vi "CC Script Parse.vi"(8 "error in (no error)":errorcluster, 11 "Script text":string="DefineObject \"Test\" Type=Standard,PositionType=RA-DEC,RA=14:25:33.123,DEC=090:15:22.110,muRA=0.000000,muDEC=0.000000,Epoch=0.000000,xi=1.000000,eta=2.000000,dRA=3.000000,dDEC=4.000000\nDefineExposure \"Standard\" Number=1,ReadoutGroups=1,ReadoutsperGroup=2,TimeBetweenGroups=10.000000,TimeBetweenReadouts=10.000000\nDefineDithering Random \"\" Count=1,Radius=1FocusMoveAbsolute Motor=1,Position=23452\nFocusMoveRelative Motor=1,Distance=23452\nAcquireImage Object=\"Test\",Exposure=\"Standard\",Dithering=\"Random\"\nFocusSetHome Motor=1\nFocusMoveRelative Motor=1,Distance=23452\nFocusMoveRelative Motor=1,Distance=23452\nTelescopeFocusHome\nTelescopeFocusMove Position=-0.123\n") -> (0 "error out":errorcluster, 1 "Syntax Errors":string, 2 "Script Ok?":bool, 3 "Script steps":T1[](array[typedef]))   [LabVIEW 2021]
uses:
  typedefs/CC Script Step.ctl
  typedefs/CC enum Script Action.ctl
  <vilib>/regexp/Match Regular Expression.xnode
panel:
  out "Errors":errorcluster[](array[cluster])
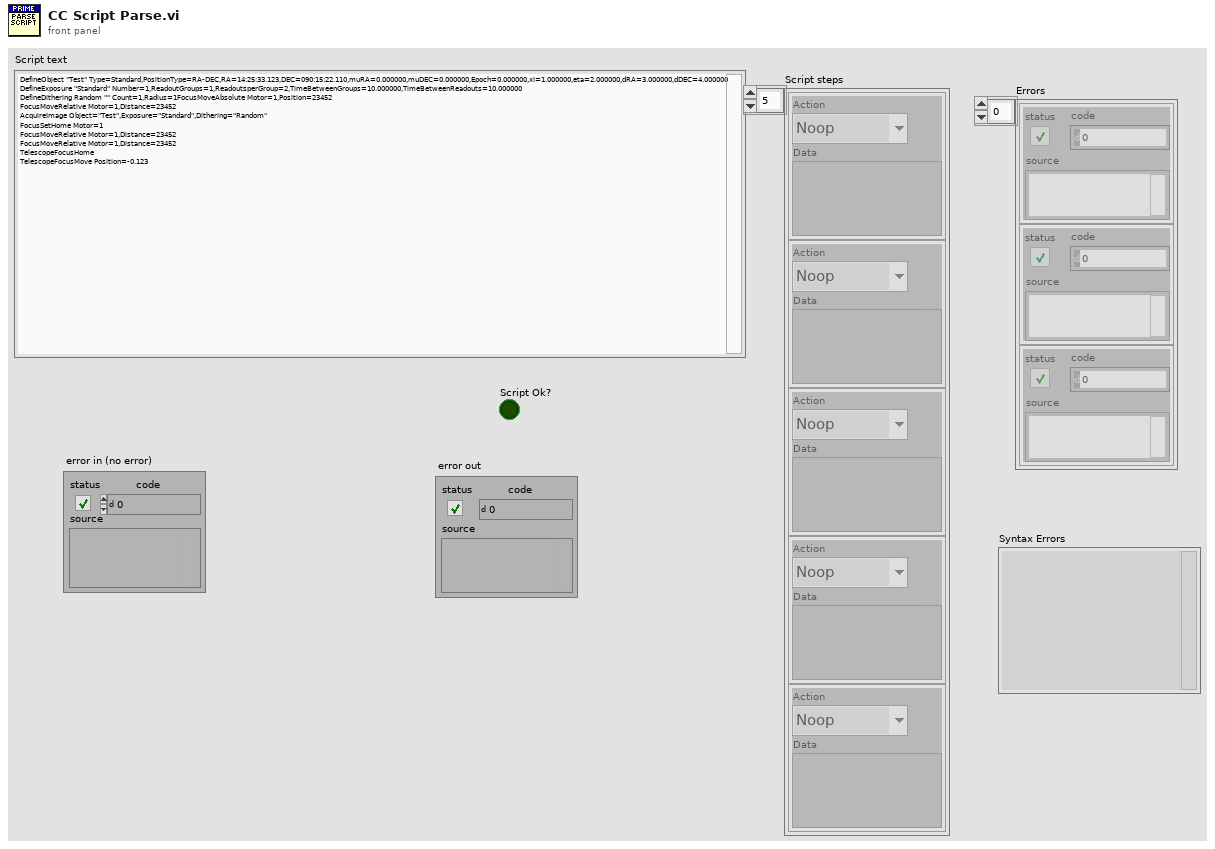
[diagram p1: front panel]
types:
  T1 = typedef "CC Script Step.ctl" = cluster{"Action":T2, "Data":variant}
  T2 = typedef "CC enum Script Action.ctl" = enum16{"Noop", "Define Object", "Define Exposure", "Define Dithering", "Acquire Images", "Set Filter Wheel", "Telescope Home", "Telescope Move", "Telescope RA DEC", "Focus Move Relative", "Focus Move Absolute", "Focus Set Home", "Macro", "Pause", "Ask User", "Define Random Dither"}
  T3 = typedef "CC cluster Object.ctl" = cluster{"Object":cluster{"Name":string}, "Sidereal Rate":T4, "RA and DEC":T5, "muRA muDEC Epoch":T6, "Offsets":T7}
  T4 = typedef "CC cluster sidereal rate.ctl" = cluster{"dRA":dbl, "dDEC":dbl}
  T5 = typedef "CC cluster RA and DEC.ctl" = cluster{"RA":dbl, "DEC":dbl}
  T6 = typedef "cc cluster muRA muDEC.ctl" = cluster{"muRA":dbl, "muDEC":dbl, "Epoch":dbl}
  T7 = typedef "CC cluster Telescope Offsets.ctl" = cluster{"RA":dbl, "DEC":dbl, "ROT":dbl}
  T8 = typedef "CC cluster Exposure.ctl" = cluster{"Mode":T9, "Integration Time":dbl, "Name":string, "Images":i32}
  T9 = typedef "Detector enum Detector Integration Mode.ctl" = enum16{"SSR", "CDS", "MEAN", "MEDIAN", "MODE", "MIIN", "MAX"}
  T10 = typedef "CC Dithering.ctl" = cluster{"Name":string, "Dithering Offsets":T11}
  T11 = typedef "CC cluster Offset Dithering.ctl" = cluster{"Offsets":T12[]}
  T12 = typedef "CC Dithering Offsets.ctl" = cluster{"DEC":dbl, "RA":dbl}
  T13 = typedef "CC cluster Random Dithering.ctl" = cluster{"Count":i32, "Radius":dbl, "Name":string}
  T14 = typedef "CC cluster Acquire Parameters.ctl" = cluster{"Object":string, "Exposure":string, "Dithering":string}
  T15 = typedef "CC cluster Filter Wheel Parameters.ctl" = cluster{"Wheel":i32, "Filter":i32}
  T16 = typedef "Focus cluster MoveFocus Command Parameters.ctl" = cluster{"Motor":i32, "Position":i32}
  T17 = typedef "CC cluster Pause Parameters.ctl" = cluster{"Time (s)":dbl}
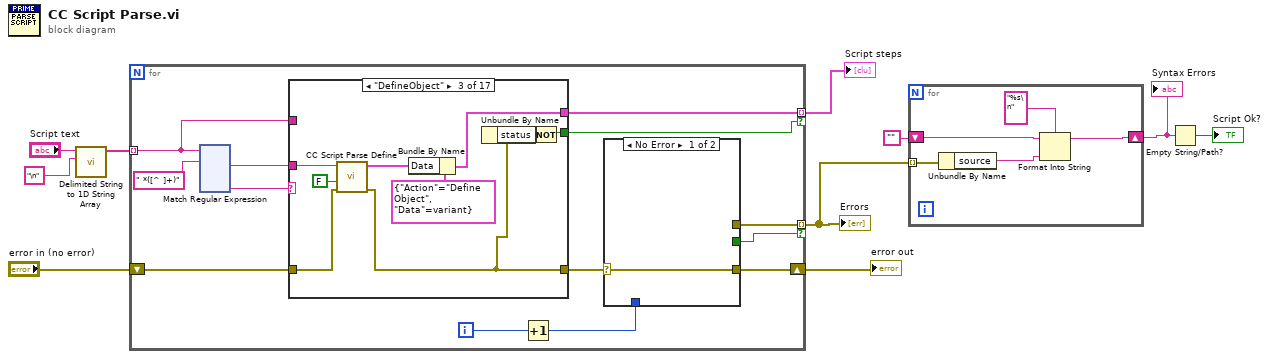
[diagram p0: block diagram]
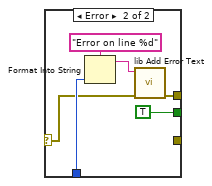
[diagram p2: hidden frame]
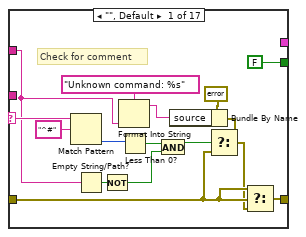
[diagram p3: hidden frame]
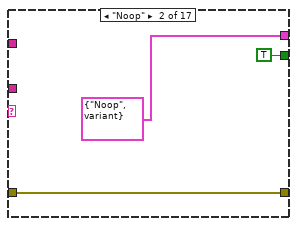
[diagram p4: hidden frame]
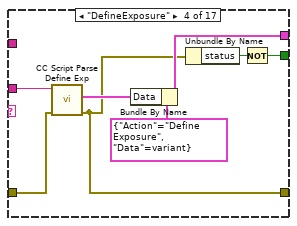
[diagram p5: hidden frame]
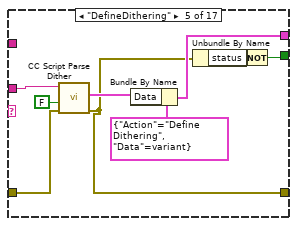
[diagram p6: hidden frame]
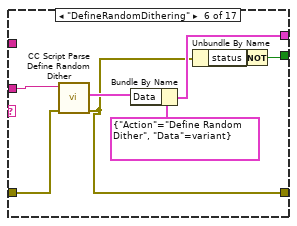
[diagram p7: hidden frame]
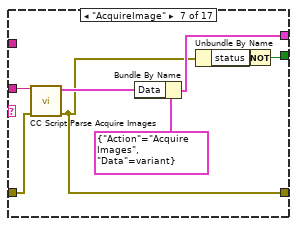
[diagram p8: hidden frame]
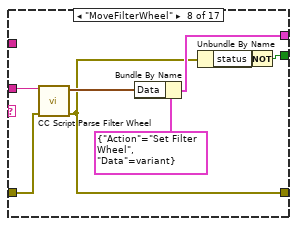
[diagram p9: hidden frame]
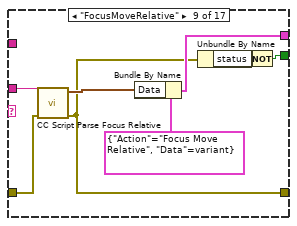
[diagram p10: hidden frame]
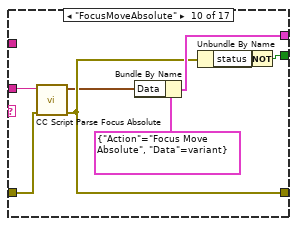
[diagram p11: hidden frame]
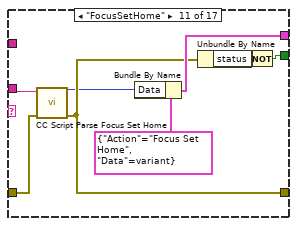
[diagram p12: hidden frame]
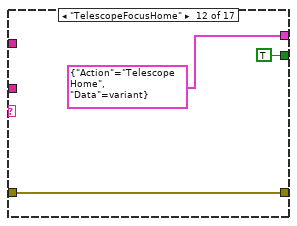
[diagram p13: hidden frame]
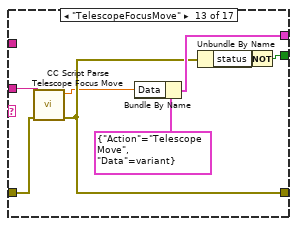
[diagram p14: hidden frame]
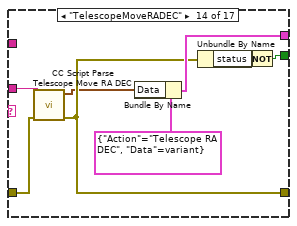
[diagram p15: hidden frame]
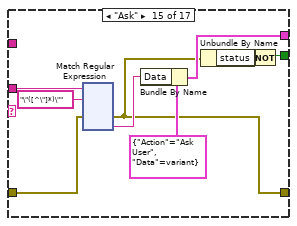
[diagram p16: hidden frame]
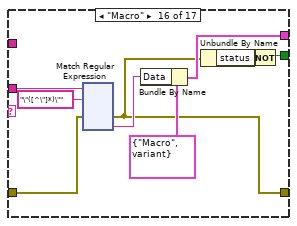
[diagram p17: hidden frame]
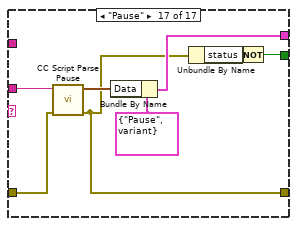
[diagram p18: hidden frame]
diagram:
  n1 = call <vilib>:"Delimited String to 1D String Array.vi"("delimiter"="\n", "delimited string"="Script text") -> ("string array"=w9:string[])  [unwired: 9 in]
  n2 = for {
    tunnel: w9 -> [w15] mode=indexing
    shift-right: [w19] -> w6
    shift-left: "error in (no error)" -> [w21]
    tunnel: [w17] -> w4 mode=indexing if=w13
    tunnel: [w14] -> w5 mode=indexing if=w12
    i -> [w18]
    n3 = xnode "Match Regular Expression"("input string"=w15, "regular expression"=" *([^ ]+)") -> ("after match"=w22:string, "submatch 1"=w11:string)  [unwired: 4 in, 4 out]
    n4 = case shown="\"DefineObject\"" w11 {
      selector: w11 -> [w36 _ _ _ _ _ _ _ _ _ _ _ _ _ _ _ _]
      tunnel: w22 -> [_ _ w58 w65 w71 w79 w90 w98 w103 w108 w119 _ w130 w138 w151 w279 w405]
      tunnel: [_ T1 {"Action"=enum."Noop", "Data"=variant} ("Cluster") w53 w62 w74 w82 w87 w95 w106 w114 w122 T1 {"Action"=enum."Telescope Home", "Data"=variant} ("Cluster") w133 w141 w146 w274 w402] -> w14
      tunnel: w21 -> [w39 w49 w56 w63 w70 w78 w88 w96 w102 w111 w118 w124 w129 w137 w147 w275 w403]
      tunnel: [w37 w49 w52 w60 w68 w76 w85 w93 w100 w110 w117 w124 w128 w136 w144 w272 w400] -> w20
      tunnel: w15 -> [w34 _ _ _ _ _ _ _ _ _ _ _ _ _ _ _ _]
      tunnel: [FALSE TRUE w50 w59 w72 w80 w84 w92 w104 w112 w120 TRUE w131 w139 w143 w271 w399] -> w12
      frame "", Default {
        # "Check for comment"
        n5 = Match Pattern(string=w36, regular expression="^#") -> (offset past match=w42:i32)  [unwired: 1 in, 3 out]
        n6 = Empty String/Path?(string/path=w34) -> (empty?=w32:bool)
        n7 = Not(x=w32) -> (.not. x?=w31:bool)
        n8 = Format Into String(format string="Unknown command: %s", w34) -> (resulting string=w43:string)  [unwired: 2 in, 1 out]
        n9 = Less Than 0?(x=w42) -> (x < 0?=w40:bool)
        n10 = And(x=w40, y=w31) -> (x .and. y?=w33:bool)
        n11 = Bundle By Name(cluster=errorcluster {"status"=TRUE, "code"=5000, "source"=""} ("error out"), "source"=w43) -> (w41:errorcluster)
        n12 = Select(t=w41, s=w33, f=w39) -> (s? t:f=w38:errorcluster)
        n13 = Select(t=w39, s=w39, f=w38) -> (s? t:f=w37:errorcluster)
      }
      frame "Noop" {
      }
      frame "DefineObject" {
        n14 = call "CC Script Parse Define.vi"("error in (no error)"=w56, "To String?"=FALSE, "DefineObject Parameters"=w58) -> ("error out"=w52:errorcluster, "Object out"=w54:T3)  [unwired: 5 in, 2 out]
        n15 = Bundle By Name(cluster=T1 {"Action"=enum."Define Object", "Data"=variant} ("Cluster"), "Data"=w54) -> (w53:T1)
        n16 = Unbundle By Name(w52) -> ("status"=w51:bool)
        n17 = Not(x=w51) -> (.not. x?=w50:bool)
      }
      frame "DefineExposure" {
        n18 = call "CC Script Parse Define Exp.vi"("error in (no error)"=w63, "DefineExp Parameters"=w65) -> ("error out"=w60:errorcluster, "Exposure"=w64:T8)  [unwired: 6 in, 2 out]
        n19 = Bundle By Name(cluster=T1 {"Action"=enum."Define Exposure", "Data"=variant} ("Cluster"), "Data"=w64) -> (w62:T1)
        n20 = Unbundle By Name(w60) -> ("status"=w61:bool)
        n21 = Not(x=w61) -> (.not. x?=w59:bool)
      }
      frame "DefineDithering" {
        n22 = call "CC Script Parse Dither.vi"("error in (no error)"=w70, "To String?"=FALSE, "Dither Parameters"=w71) -> ("error out"=w68:errorcluster, "Dithering out"=w69:T10)  [unwired: 6 in, 1 out]
        n23 = Bundle By Name(cluster=T1 {"Action"=enum."Define Dithering", "Data"=variant} ("Cluster"), "Data"=w69) -> (w74:T1)
        n24 = Unbundle By Name(w68) -> ("status"=w73:bool)
        n25 = Not(x=w73) -> (.not. x?=w72:bool)
      }
      frame "DefineRandomDithering" {
        n26 = call "CC Script Parse Define Random Dither.vi"("error in (no error)"=w78, "Dither Parameters"=w79) -> ("error out"=w76:errorcluster, "Random Dither out"=w77:T13)  [unwired: 7 in, 1 out]
        n27 = Bundle By Name(cluster=T1 {"Action"=enum."Define Random Dither", "Data"=variant} ("Cluster"), "Data"=w77) -> (w82:T1)
        n28 = Unbundle By Name(w76) -> ("status"=w81:bool)
        n29 = Not(x=w81) -> (.not. x?=w80:bool)
      }
      frame "AcquireImage" {
        n30 = call "CC Script Parse Acquire Images.vi"("error in (no error)"=w88, "DefineObject Parameters"=w90) -> ("error out"=w85:errorcluster, "Acquire Parameters"=w89:T14)  [unwired: 7 in, 1 out]
        n31 = Bundle By Name(cluster=T1 {"Action"=enum."Acquire Images", "Data"=variant} ("Cluster"), "Data"=w89) -> (w87:T1)
        n32 = Unbundle By Name(w85) -> ("status"=w86:bool)
        n33 = Not(x=w86) -> (.not. x?=w84:bool)
      }
      frame "MoveFilterWheel" {
        n34 = call "CC Script Parse Filter Wheel.vi"("error in (no error)"=w96, "DefineObject Parameters"=w98) -> ("error out"=w93:errorcluster, "Filter Wheel Parameters"=w97:T15)  [unwired: 7 in, 1 out]
        n35 = Bundle By Name(cluster=T1 {"Action"=enum."Set Filter Wheel", "Data"=variant} ("Cluster"), "Data"=w97) -> (w95:T1)
        n36 = Unbundle By Name(w93) -> ("status"=w94:bool)
        n37 = Not(x=w94) -> (.not. x?=w92:bool)
      }
      frame "FocusMoveRelative" {
        n38 = call "CC Script Parse Focus Relative.vi"("error in (no error)"=w102, "DefineObject Parameters"=w103) -> ("error out"=w100:errorcluster, "Filter Wheel parameters in"=w101:T16)  [unwired: 7 in, 1 out]
        n39 = Bundle By Name(cluster=T1 {"Action"=enum."Focus Move Relative", "Data"=variant} ("Cluster"), "Data"=w101) -> (w106:T1)
        n40 = Unbundle By Name(w100) -> ("status"=w105:bool)
        n41 = Not(x=w105) -> (.not. x?=w104:bool)
      }
      frame "FocusMoveAbsolute" {
        n42 = call "CC Script Parse Focus Absolute.vi"("error in (no error)"=w111, "FocusMoveAbsolute Parameters"=w108) -> ("error out"=w110:errorcluster, "Filter Wheel parameters in"=w109:T16)  [unwired: 7 in, 1 out]
        n43 = Bundle By Name(cluster=T1 {"Action"=enum."Focus Move Absolute", "Data"=variant} ("Cluster"), "Data"=w109) -> (w114:T1)
        n44 = Unbundle By Name(w110) -> ("status"=w113:bool)
        n45 = Not(x=w113) -> (.not. x?=w112:bool)
      }
      frame "FocusSetHome" {
        n46 = call "CC Script Parse Focus Set Home.vi"("error in (no error)"=w118, "DefineObject Parameters"=w119) -> ("error out"=w117:errorcluster, "Set Home Parm"=w116:i32)  [unwired: 7 in, 1 out]
        n47 = Bundle By Name(cluster=T1 {"Action"=enum."Focus Set Home", "Data"=variant} ("Cluster"), "Data"=w116) -> (w122:T1)
        n48 = Unbundle By Name(w117) -> ("status"=w121:bool)
        n49 = Not(x=w121) -> (.not. x?=w120:bool)
      }
      frame "TelescopeFocusHome" {
      }
      frame "TelescopeFocusMove" {
        n50 = call "CC Script Parse Telescope Focus Move.vi"("error in (no error)"=w129, "Telescope Move Parameters"=w130) -> ("error out"=w128:errorcluster, "Telescope Move Pos"=w127:dbl)  [unwired: 7 in, 1 out]
        n51 = Bundle By Name(cluster=T1 {"Action"=enum."Telescope Move", "Data"=variant} ("Cluster"), "Data"=w127) -> (w133:T1)
        n52 = Unbundle By Name(w128) -> ("status"=w132:bool)
        n53 = Not(x=w132) -> (.not. x?=w131:bool)
      }
      frame "TelescopeMoveRADEC" {
        n54 = call "CC Script Parse Telescope Move RA DEC.vi"("error in (no error)"=w137, "Telescope Move Parameters"=w138) -> ("error out"=w136:errorcluster, "RA and DEC"=w135:T5)  [unwired: 7 in, 1 out]
        n55 = Bundle By Name(cluster=T1 {"Action"=enum."Telescope RA DEC", "Data"=variant} ("Cluster"), "Data"=w135) -> (w141:T1)
        n56 = Unbundle By Name(w136) -> ("status"=w140:bool)
        n57 = Not(x=w140) -> (.not. x?=w139:bool)
      }
      frame "Ask" {
        n58 = xnode "Match Regular Expression"("input string"=w151, "regular expression"="\"([^\"]*)\"", "error in"=w147) -> ("error out"=w144:errorcluster, "submatch 1"=w148:string)  [unwired: 3 in, 4 out]
        n59 = Bundle By Name(cluster=T1 {"Action"=enum."Ask User", "Data"=variant} ("Cluster"), "Data"=w148) -> (w146:T1)
        n60 = Unbundle By Name(w144) -> ("status"=w145:bool)
        n61 = Not(x=w145) -> (.not. x?=w143:bool)
      }
      frame "Macro" {
        n62 = xnode "Match Regular Expression"("input string"=w279, "regular expression"="\"([^\"]*)\"", "error in"=w275) -> ("error out"=w272:errorcluster, "submatch 1"=w276:string)  [unwired: 3 in, 4 out]
        n63 = Bundle By Name(cluster=T1 {"Action"=enum."Macro", "Data"=variant} ("Cluster"), "Data"=w276) -> (w274:T1)
        n64 = Unbundle By Name(w272) -> ("status"=w273:bool)
        n65 = Not(x=w273) -> (.not. x?=w271:bool)
      }
      frame "Pause" {
        n66 = call "CC Script Parse Pause.vi"("error in (no error)"=w403, "DefineObject Parameters"=w405) -> ("error out"=w400:errorcluster, "Pause Parameters"=w404:T17)  [unwired: 8 in]
        n67 = Bundle By Name(cluster=T1 {"Action"=enum."Pause", "Data"=variant} ("Cluster"), "Data"=w404) -> (w402:T1)
        n68 = Unbundle By Name(w400) -> ("status"=w401:bool)
        n69 = Not(x=w401) -> (.not. x?=w399:bool)
      }
    }
    n70 = Increment(x=w18) -> (x+1=w16:i32)
    n71 = case shown="No Error" w20 {
      selector: w20 -> [w24 w28]
      tunnel: [w24 _] -> w19
      tunnel: w16 -> [_ w29]
      tunnel: [_ w26] -> w17
      tunnel: [_ TRUE] -> w13
      frame No Error {
      }
      frame Error {
        n72 = Format Into String(format string="Error on line %d", w29) -> (resulting string=w27:string)  [unwired: 2 in, 1 out]
        n73 = call "lib Add Error Text.vi"("error in (no error)"=w28, "Append to source, if error"=w27) -> ("error out"=w26:errorcluster)  [unwired: 9 in]
      }
    }
  }
  "error out" <- w6
  "Script steps" <- w5
  "Errors" <- w4
  n74 = for {
    tunnel: w4 -> [w530] mode=indexing
    shift-right: [w526] -> w2
    shift-left: "" -> [w529]
    n75 = Unbundle By Name(w530) -> ("source"=w527:string)
    n76 = Format Into String(format string="%s\n", initial string=w529, w527) -> (resulting string=w526:string)  [unwired: 1 in, 1 out]
  }
  "Syntax Errors" <- w2
  n77 = Empty String/Path?(string/path=w2) -> (empty?=→"Script Ok?":bool)
